vi "Read Single Encoder.vi"(9 "TC":dbl, 10 "Rate":dbl, 11 "Distance":dbl) -> (3 "Single Encoder Data 2":T1)   [LabVIEW 2015]
uses:
  Single Encoder Data.ctl
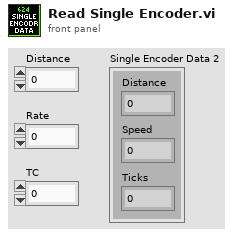
[diagram p1: front panel]
types:
  T1 = typedef "Single Encoder Data.ctl" = cluster{"Distance":dbl, "Speed":dbl, "Ticks":dbl}
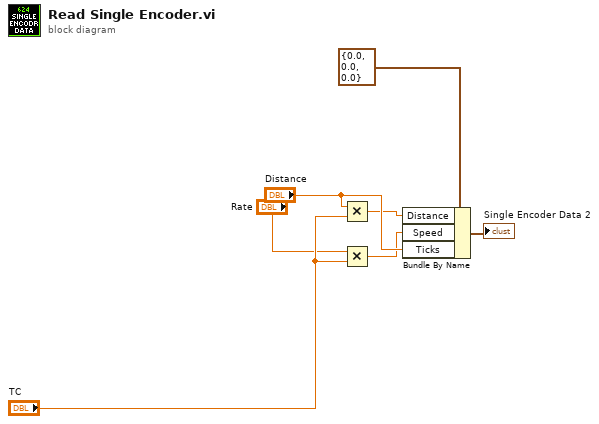
[diagram p0: block diagram]
diagram:
  n1 = Multiply(x="Distance", y="TC") -> (x*y=w5:dbl)
  n2 = Multiply(x="Rate", y="TC") -> (x*y=w6:dbl)
  n3 = Bundle By Name(cluster=T1 {"Distance"=0.0, "Speed"=0.0, "Ticks"=0.0} ("Single Encoder Data 2"), "Distance"=w5, "Speed"=w6, "Ticks"="Distance") -> (→"Single Encoder Data 2":T1)
